vi "Start Recording.vi"(8 "error in (no error)":errorcluster, 10 "Protocol":refnum<class "Protocol.lvclass">, 11 "Application in":refnum<class "Application.lvclass">) -> (0 "error out":errorcluster, 3 "Application out":refnum<class "Application.lvclass">)   [LabVIEW 2023, in "Application.lvlib" / "Application.lvclass"]
uses:
  Application.lvclass
  Automation/Protocol/Protocol.lvclass
  Application.lvclass/Application.ctl
  Mode.ctl
  User Interface/Main Window Messages/Application Mode Change Msg/Application Mode Change Msg.lvclass/Application Mode Change Msg.ctl
  <vilib>/ActorFramework/Message Enqueuer/Message Enqueuer.lvclass/Message Enqueuer.ctl
  <vilib>/ActorFramework/Message Enqueuer/Enqueue.vi
  User Interface/Main Window Messages/Application Mode Change Msg/Application Mode Change Msg.lvclass
  <vilib>/ActorFramework/Message Priority Queue/Priority Enqueue.vi
  Application.lvlib
  Automation/AutomationContext.lvclass
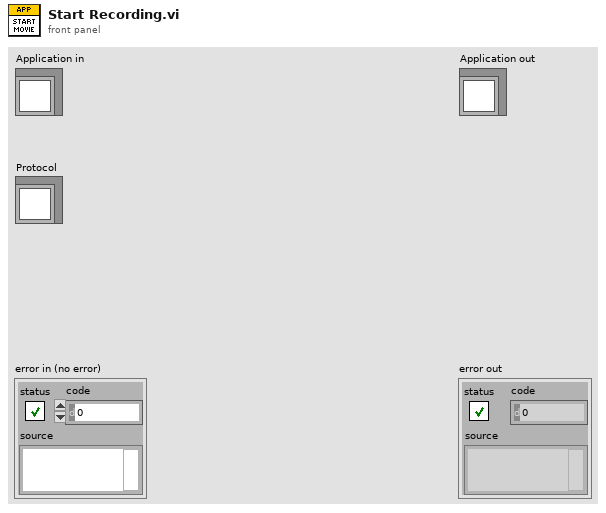
[diagram p1: front panel]
types:
  T1 = typedef "Application.lvlib/Mode.ctl" = enum16{"Idle", "Cancel", "Live", "Stream", "Autofocus", "Z-Stack", "Montage", "Saving", "Stage Scan", "Laser Adjust"}
  T2 = typedef "Hardware Configuration.ctl" = cluster{"Stage Configuration":T3, "Microscope Configuration":T4, "Virtual Camera Configuration":T6, "Laser Configuration":T8[], "Installed Cameras":T9[], "Power Meter Configuration":cluster{"Power Meter Type":enum16{"Disabled", "Thorlabs", "Newport", "Coherent"}, "attenuation":dbl, "instrument handle":refnum<visa-resource-name>}, "DAQ Configuration":T10}
  T3 = typedef "Stage Configuration.ctl" = cluster{"Serial Port":refnum<visa-resource-name>, "Forward Step (mm)":dbl, "Lane Length (mm)":dbl, "Lane Separation (mm)":dbl, "Stage Type":enum16{"Disabled", "ESP301", "Ti2", "Ludl", "ASI", "Simulate"}, "Autofocus Z Planes":i32, "Autofocus Range (um)":dbl, "Stage Limits":cluster{"Y Min":dbl, "Y Max":dbl, "X Min":dbl, "X Max":dbl}, "Slide (mm)":cluster{"top":dbl, "right":dbl, "width":dbl, "height":dbl}}
  T4 = typedef "Microscope Configuration.ctl" = cluster{"Serial Port":refnum<visa-resource-name>, "Microscope Type":T5, "Detection Settings":cluster{"Name":string, "Filter Position":u16, "Optical Path":u16}[]}
  T5 = typedef "Microscope Type.ctl" = enum16{"Disable", "TE2000", "Eclipse Ti", "Ti2"}
  T6 = typedef "Virtual Camera Configuration.ctl" = cluster{"Camera Type":T7}
  T7 = typedef "Camera Type.ctl" = enum16{"Hamamatsu", "Andor", "Photometrics"}
  T8 = typedef "Laser Configuration.ctl" = cluster{"Serial Port":refnum<visa-resource-name>, "Laser Type":enum16{"Disable", "Laser Quantum", "Coherent OBIS", "PRM1-Z8", "Coherent HOPS", "Cobolt"}, "Polarizer Amplitude":dbl, "Polarizer Theta Zero":dbl, "Wavelength":u16}
  T9 = typedef "Physical Camera Assignment.ctl" = cluster{"Channel Name":string, "Serial Number":string, "Flip Vertically":bool, "Flip Horizontally":bool, "wavelength":i16, "photonsPerCount":dbl[]}
  T10 = typedef "DAQ Configuration.ctl" = cluster{"Shutters":T11[], "fluidics trigger line":tag, "camera trigger line":tag, "COM Port":refnum<visa-resource-name>, "Device type":T12}
  T11 = typedef "Shutter Configuration.ctl" = cluster{"IO Line":tag, "Name":string, "Wavelength":u16, "Max rate (Hz)":dbl}
  T12 = typedef "Sync Device Type.ctl" = enum16{"Disabled", "NI DAQ", "Arduino DAQ", "Microsync"}
  T13 = typedef "Camera Settings.ctl" = cluster{"Exposure Time (ms)":dbl, "Binning":enum16{"1x1", "2x2", "4x4"}, "Scan Mode":i32, "Frames to Acquire":dbl, "Pixel Correction":bool, "Frames to Skip":u32, "File Path":path, "Duty cycle":dbl, "ALEX":bool, "Shutter Enable":bool[], "fluidics trigger, ms (0=disabled)":dbl, "Bit Depth":u16, "Image Width (px)":u16, "Image Height (px)":u16, "Horizontal Offset (px)":u16, "Vertical Offset (px)":u16}
  T14 = typedef "Movie auto-numbering.ctl" = enum16{"Single movie", "Movie series", "Multi-lane series"}
  T15 = cluster{"Camera Settings":T13, "Auto-Advance":bool, "Auto Focus":bool, "Injection Countdown":bool, "Fields":i32, "Lanes":i32, "Acquisition type":T14, "Particle Count Threshold":i32}
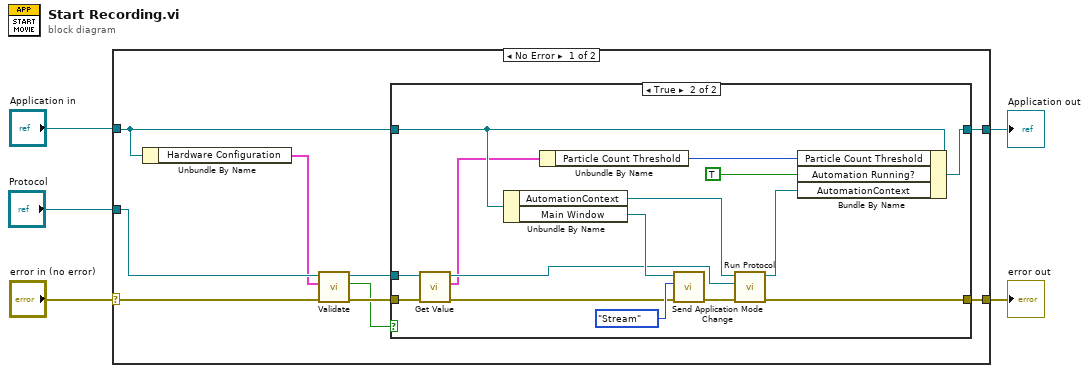
[diagram p0: block diagram]
diagram:
  n1 = case shown="No Error" "error in (no error)" {
    selector: "error in (no error)" -> [w12 w33]
    tunnel: [w13 w33] -> w4
    tunnel: [w14 w32] -> w2
    tunnel: "Application in" -> [w10 w32]
    tunnel: "Protocol" -> [w11 _]
    frame No Error {
      n2 = Unbundle By Name(w10) -> ("Hardware Configuration"=w9:T2)
      n3 = call "Validate.vi"("error in (no error)"=w12, "Hardware Configuration"=w9, "Protocol in"=w11) -> ("error out"=w8:errorcluster, "Ok?"=w7:bool, "Protocol out"=w6:refnum<class "Protocol.lvclass">)  [unwired: 6 in]
      n4 = case shown="True" w7 {
        tunnel: w8 -> [w15 w21]
        tunnel: [w16 w31] -> w14
        tunnel: w10 -> [w16 w30]
        tunnel: [w15 w24] -> w13
        tunnel: w6 -> [_ w20]
        frame False {
        }
        frame True {
          n5 = call "Get Value.vi"("error in (no error)"=w21, "Protocol in"=w20) -> ("error out"=w19:errorcluster, "Movie Series"=w17:T15, "Protocol out"=w18:refnum<class "Protocol.lvclass">)  [unwired: 7 in]
          n6 = Unbundle By Name(w30) -> ("AutomationContext"=w23:refnum<class "AutomationContext.lvclass">, "Main Window"=w28:refnum<class "Message Enqueuer.lvclass">)
          n7 = Unbundle By Name(w17) -> ("Particle Count Threshold"=w26:i32)
          n8 = call "Send Application Mode Change.vi"("error in (no error)"=w19, "Mode"=Mode."Stream", "Message Enqueuer"=w28) -> ("error out"=w25:errorcluster)  [unwired: 7 in, 1 out]
          n9 = call "Run Protocol.vi"("error in (no error)"=w25, "Protocol"=w18, "AutomationContext in"=w23) -> ("error out"=w24:errorcluster, "AutomationContext out"=w22:refnum<class "AutomationContext.lvclass">)  [unwired: 7 in]
          n10 = Bundle By Name(cluster=w30, "Particle Count Threshold"=w26, "Automation Running?"=TRUE, "AutomationContext"=w22) -> (w31:refnum<class "Application.lvclass">)
        }
      }
    }
    frame Error {
    }
  }
  "error out" <- w4
  "Application out" <- w2
